vi "Lift.vi"(9 "Up Button":bool, 10 "Down Button":bool, 11 "Solenoid Ref Name":string="My Solenoid RefNum") -> (3 "Lift Motor":dbl)   [LabVIEW 2014]
uses:
  <vilib>/Rock Robotics/WPI/Solenoid/WPI_SolenoidValue.ctl
  <vilib>/Rock Robotics/WPI/Solenoid/WPI_SolenoidSetEnum.vi
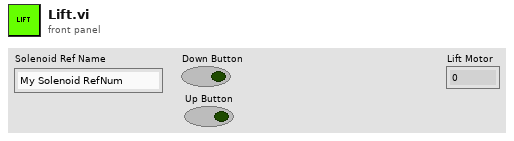
[diagram p1: front panel]
types:
  T1 = typedef "WPI_SolenoidDevRef.ctl" = cluster{"DevStatus":errorcluster, "Pneumatics Control Module":u8, "Forward Solenoid Channel":T2, "Reverse Solenoid Channel":T2}
  T2 = typedef "WPI_SolenoidChannel.ctl" = enum8{"Solenoid 0", "Solenoid 1", "Solenoid 2", "Solenoid 3", "Solenoid 4", "Solenoid 5", "Solenoid 6", "Solenoid 7", "Invalid"}
  T3 = typedef "WPI_SolenoidValue.ctl" = enum16{"Off", "On", "Forward", "Reverse"}
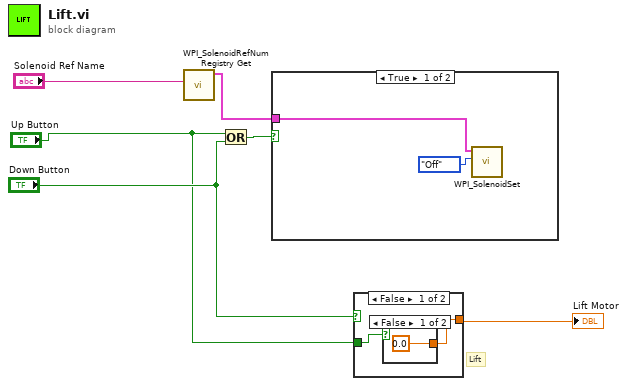
[diagram p0: block diagram]
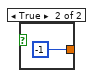
[diagram p2: hidden frame]
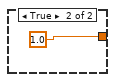
[diagram p3: hidden frame]
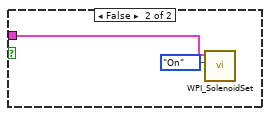
[diagram p4: hidden frame]
diagram:
  # "Lift"
  n1 = call <vilib>:"WPI_SolenoidRefNum Registry Get.vi"("refnum name"="Solenoid Ref Name") -> ("SolenoidDevRef"=w2:T1)  [unwired: 9 in, 1 out]
  n2 = Or(x="Up Button", y="Down Button") -> (x .or. y?=w5:bool)
  n3 = case shown="True" w5 {
    tunnel: w2 -> [w7 w10]
    frame True {
      n4 = call-poly <vilib>:"WPI_SolenoidSet.vi"("Value"=WPI_SolenoidValue."Off", "SolenoidDevRef"=w7) -> ()  [unwired: 8 in, 2 out]
    }
    frame False {
      n5 = call-poly <vilib>:"WPI_SolenoidSet.vi"("Value"=WPI_SolenoidValue."On", "SolenoidDevRef"=w10) -> ()  [unwired: 8 in, 2 out]
    }
  }
  n6 = case shown="False" "Down Button" {
    tunnel: [w12 1.0 ("f")] -> w6
    tunnel: "Up Button" -> [w11 _]
    frame False {
      n7 = case shown="False" w11 {
        tunnel: [0.0 -1] -> w12
        frame False {
        }
        frame True {
        }
      }
    }
    frame True {
    }
  }
  "Lift Motor" <- w6
